vi "Tension.vi"() -> ()   [LabVIEW 2015]
panel:
  in  "stop":bool
  out "Alarma Nivel\nInferior":bool=TRUE
  in  "Ref. Min":dbl=113.0
  out "Alarma Nivel\nSuperior":bool
  in  "Ref. Max":dbl=119.0
  out "Min value":dbl=112.84418138411287
  out "Max value":dbl=115.21464133659367
  out "Valores en\nMemoria":dbl[](array[numeric])=[115.21464133659367, 113.77404109406774, 113.52242999917594, 112.84418138411287, 113.13991880245788]
  out "Ultimo Valor de\nla Iteracion":dbl=113.13991880245788
  in  "Tiempo de Procesamiento\nen Milisegundos":u32=100
  in  "No. de Lecturas\nen el Arreglo":i32=5
  out "Tension\nPromedio":cluster{dbl, dbl}(graph)={112.77940874621227, 111.05655996290392}
  out "Valor Instantaneo\nde Tension":dbl=111.05655996290392
  # "Sistema de Supervison de tensión"
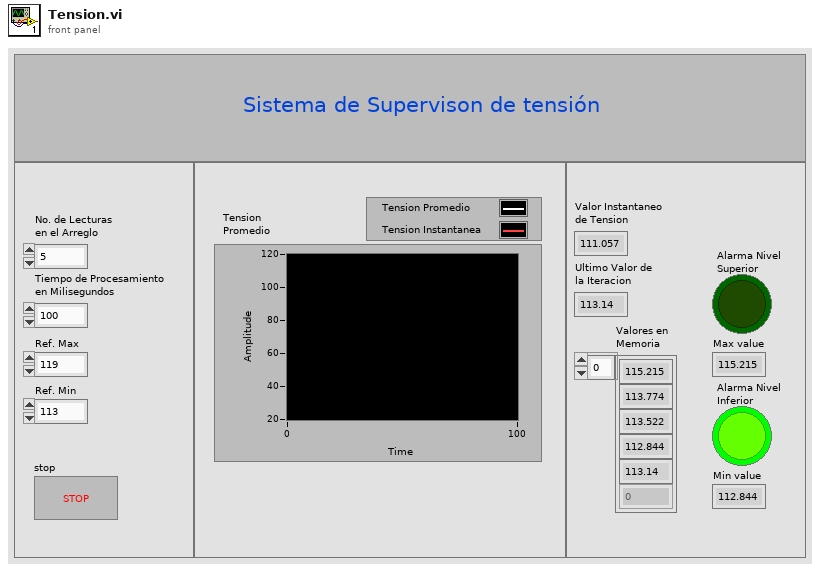
[diagram p1: front panel]
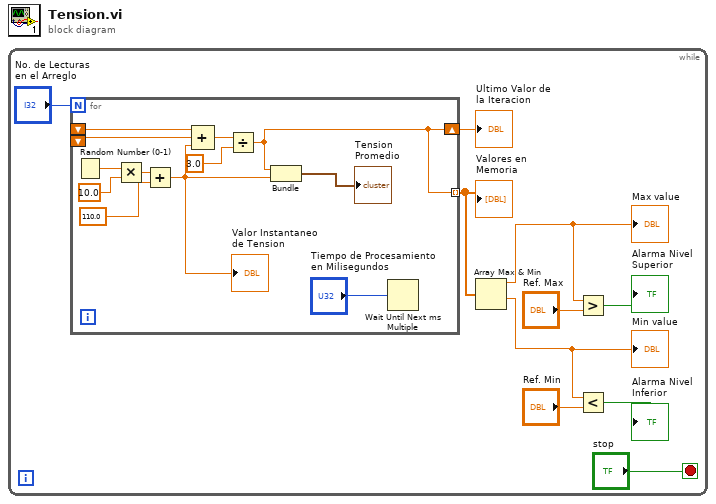
[diagram p0: block diagram]
diagram:
  n1 = while {
    stop <- "stop" stop-if-true
    n2 = for {
      N: "No. de Lecturas\nen el Arreglo" -> [_]
      shift-right: [w11] -> w9
      shift-left: _ -> [w14]
      shift-left: _ -> [w13]
      tunnel: [w11] -> w8 mode=indexing
      n3 = Random Number (0-1)() -> (number: 0 to 1=w22:dbl)
      n4 = Multiply(x=w22, y=10.0) -> (x*y=w20:dbl)
      n5 = Add(x=w20, y=110.0) -> (x+y=w18:dbl)
      "Valor Instantaneo\nde Tension" <- w18
      n6 = Compound Arithmetic op=ADD(w14, w13, w18) -> (w17:dbl)
      n7 = Divide(x=w17, y=3.0) -> (x/y=w11:dbl)
      n8 = Bundle(w11, w18) -> (→"Tension\nPromedio":cluster{dbl, dbl})  [unwired: 1 in]
      n9 = Wait Until Next ms Multiple(millisecond multiple="Tiempo de Procesamiento\nen Milisegundos") -> ()  [unwired: 1 out]
    }
    "Ultimo Valor de\nla Iteracion" <- w9
    "Valores en\nMemoria" <- w8
    n10 = Array Max & Min(array=w8) -> (max value=w7:dbl, min value=w4:dbl)  [unwired: 2 out]
    "Max value" <- w7
    "Min value" <- w4
    n11 = Greater?(x=w7, y="Ref. Max") -> (0:→"Alarma Nivel\nSuperior":bool)
    n12 = Less?(x=w4, y="Ref. Min") -> (x < y?=→"Alarma Nivel\nInferior":bool)
  }
